vi "water pressure sensor fgv.vi"(7 "Command":T1, 8 "error constant":errorcluster, 10 "Sprinkler Cmd Data Cluster":u32) -> (0 "error IO":errorcluster, 3 "Sprinkler Cmd Data Cluster":u32)   [LabVIEW 2013]
doc: "This Sub VI is use to set data and get data"
uses:
  water pressuer sensor fgv.ctl
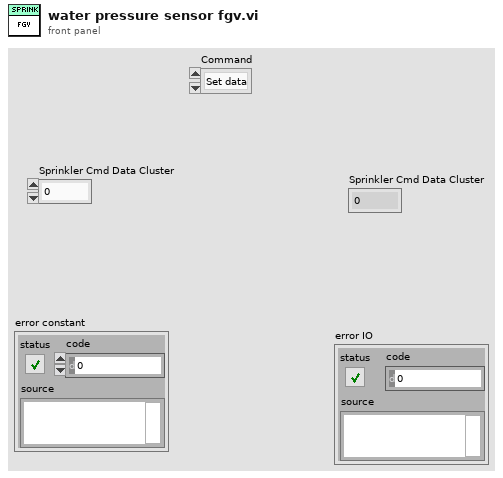
[diagram p1: front panel]
types:
  T1 = typedef "water pressuer sensor fgv.ctl" = enum16{"Set data ", "Get data"}
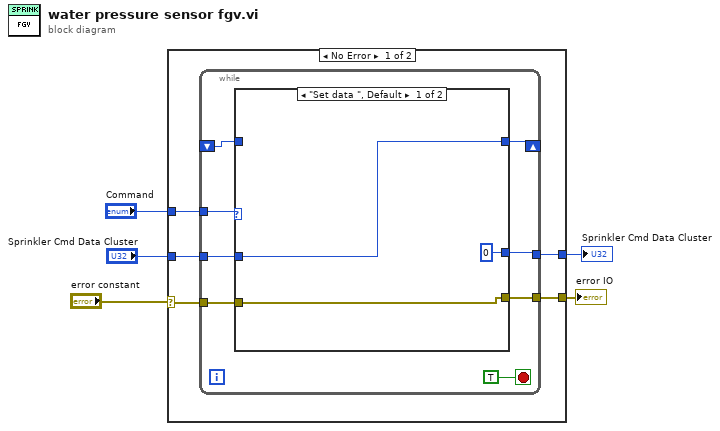
[diagram p0: block diagram]
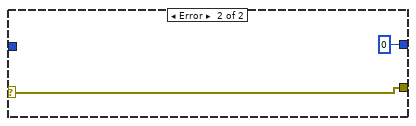
[diagram p3: hidden frame]
diagram:
  n1 = case shown="No Error" "error constant" {
    selector: "error constant" -> [w7 w24]
    tunnel: [w10 0 ("Numeric in")] -> w5
    tunnel: "Sprinkler Cmd Data Cluster" -> [w9 _]
    tunnel: "Command" -> [w8 _]
    tunnel: [w6 w24] -> w1
    frame No Error {
      n2 = while {
        tunnel: w8 -> [w18]
        tunnel: w9 -> [w17]
        shift-right: [w16] -> _
        shift-left: _ -> [w15]
        tunnel: [w14] -> w10
        tunnel: w7 -> [w13]
        tunnel: [w12] -> w6
        stop <- TRUE stop-if-true
        n3 = case shown="\"Set data \", Default" w18 {
          tunnel: w17 -> [w21 _]
          tunnel: [w21 w23] -> w16
          tunnel: w15 -> [_ w23]
          tunnel: [0 ("Numeric in") w23] -> w14
          tunnel: w13 -> [w20 w22]
          tunnel: [w20 w22] -> w12
          frame "Set data ", Default {
          }
          frame "Get data" {
          }
        }
      }
    }
    frame Error {
    }
  }
  "Sprinkler Cmd Data Cluster" <- w5
  "error IO" <- w1
